vi "PWRVT_Multi_thread.vi"() -> ()   [LabVIEW 2017]
doc: "Use this template to build a producer/consumer design pattern. Use this template when you need to execute a process, such as data analysis, when a data source, such as a triggered acquisition, produces data at an uneven rate and you need to execute the process when the data becomes available."
uses:
  ModbusRTU/Process/Process.lvclass
  ModbusRTU/Caculator/Caculator.lvclass
  ModbusRTU/LNAX301/LNAX301.lvclass
  ModbusRTU/ModbusRTUCmd.ctl
  ModbusRTU/Process/Process.ctl
  ModbusRTU/Caculator/Caculator.ctl
  DLL/Modbus.dll
panel:
  out "connect":bool
  in  "switch":bool
  in  "Debug":bool
  in  "stop":bool
  in  "Tab Control":enum32{"Main", "OA"}(tab)
  out "COM Port":string
  out "Waveform Graph":waveform(dbl)[](graph)
  out "SN":string
  in  "HPF enable":bool
  in  "軸向選擇":enum16{"X", "Y", "Z"}(ring)=enum."Z"
  out "X-Axis Peak(Vel)":dbl
  out "Y-Axis Peak(Vel)":dbl
  out "Z-Axis Peak(Vel)":dbl
  out "X-Axis RMS(Vel)":dbl
  out "Y-Axis RMS(Vel)":dbl
  out "Z-Axis RMS(Vel)":dbl
  out "X-Axis CF(ACC)":dbl
  out "Y-Axis CF(ACC)":dbl
  out "Z-Axis CF(ACC)":dbl
  out "X-Axis RMS(ACC)":dbl
  out "Y-Axis RMS(ACC)":dbl
  out "Z-Axis RMS(ACC)":dbl
  out "X-Axis Peak(ACC)":dbl
  out "Y-Axis Peak(ACC)":dbl
  out "Z-Axis Peak(ACC)":dbl
  out "Z-Axis CF(Vel)":dbl
  out "Y-Axis CF(Vel)":dbl
  out "X-Axis CF(Vel)":dbl
  out "error out 2":errorcluster
  in  "Serial Setting":T1={"baudRate"=3000000, "parity"=0, "dataBits"=8, "stopBits"=1} {"stopBits" items=["None", "One", "Two", "OnePointFive"]; "parity" items=["None", "Odd", "Even", "Mark", "Space"]}
  in  "SR":u16=7812
  # "OA Mode"
  # "Timewave Mode"
  # "HPF:需再開始量測前就決定是否開啟"
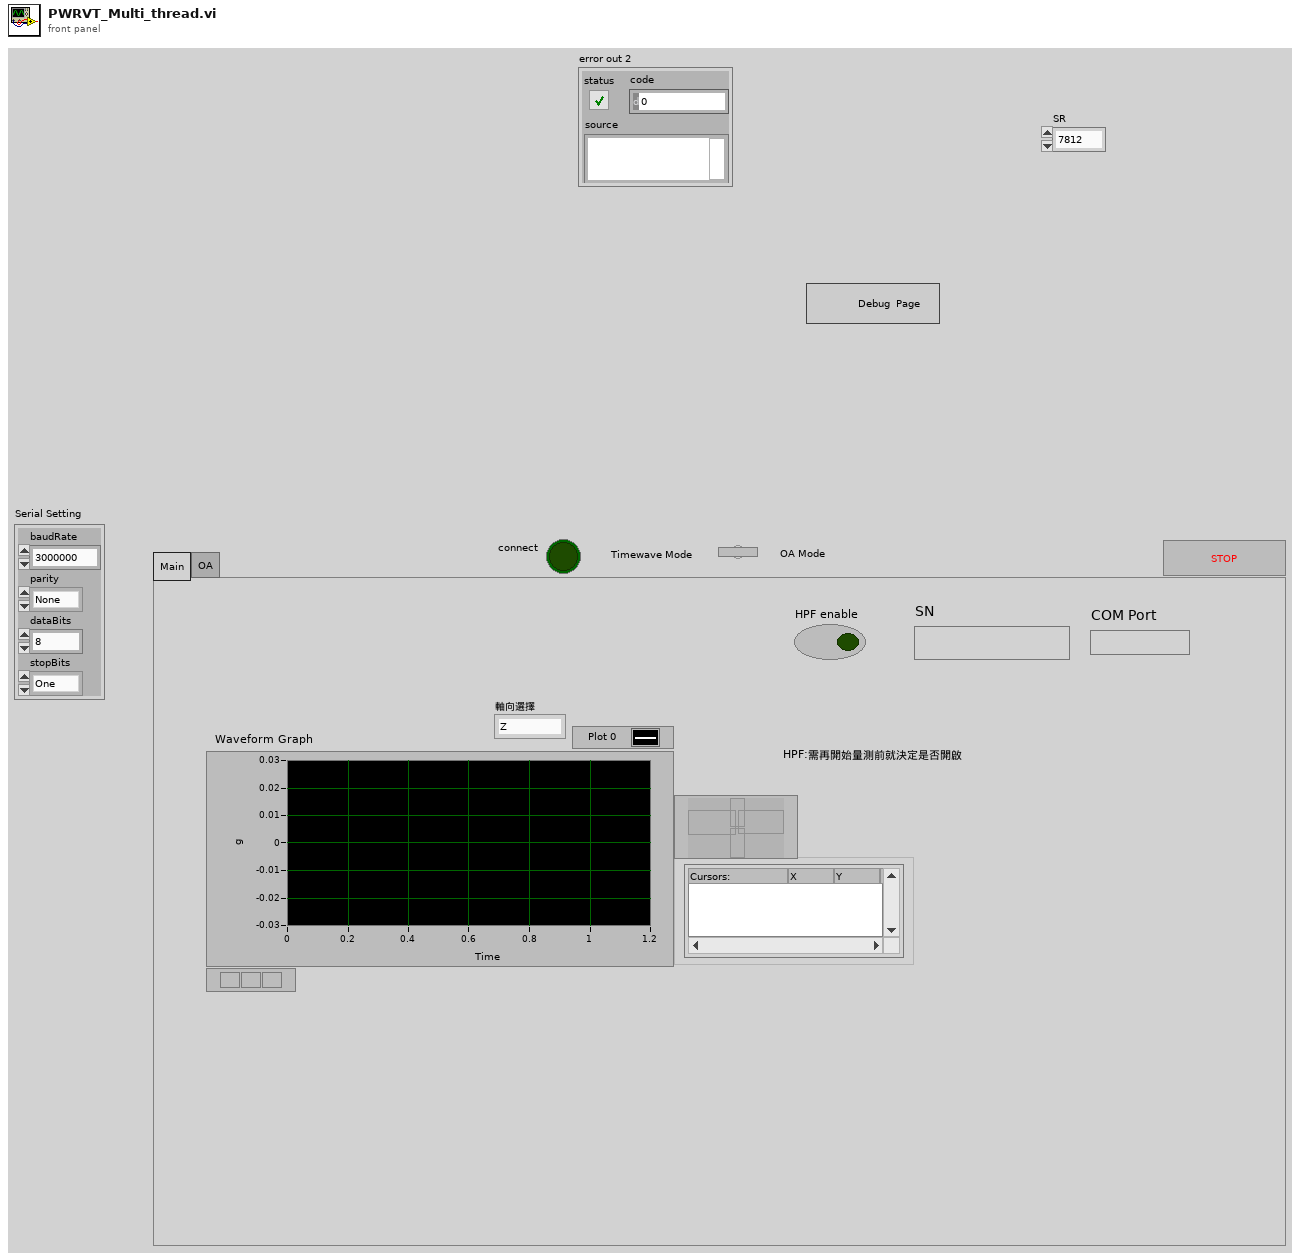
[diagram p1: front panel]
types:
  T1 = cluster{"baudRate":i32, "parity":i32, "dataBits":i32, "stopBits":i32}
  T2 = typedef "MEMS.ctl" = cluster{"LNAX301":refnum<queue>, "Process":refnum<queue>, "Caculator":refnum<queue>}
  T3 = typedef "ModbusRTUCmd.ctl" = cluster{"CMD":enum16{"Idle", "ini", "Connect", "Setup", "Read", "Disconnect", "Exit"}, "Var":variant}
  T4 = typedef "Process.ctl" = cluster{"cmd":enum16{"Idle", "ini", "CheckData", "Disconnect", "UpdateSetup", "UpdateInstance", "Exit"}, "Var":variant}
  T5 = enum16{"Idle", "ini", "Connect", "Setup", "Read", "Disconnect", "Exit"}
  T6 = enum16{"Idle", "ini", "CheckData", "Disconnect", "UpdateSetup", "UpdateInstance", "Exit"}
  T7 = typedef "Caculator.ctl" = cluster{"cmd":enum16{"Idle", "ini", "Disconnect", "UpdateSetup", "ChangeView", "Caculator", "Exit"}, "Var":variant}
  T8 = enum16{"Idle", "ini", "Disconnect", "UpdateSetup", "ChangeView", "Caculator", "Exit"}
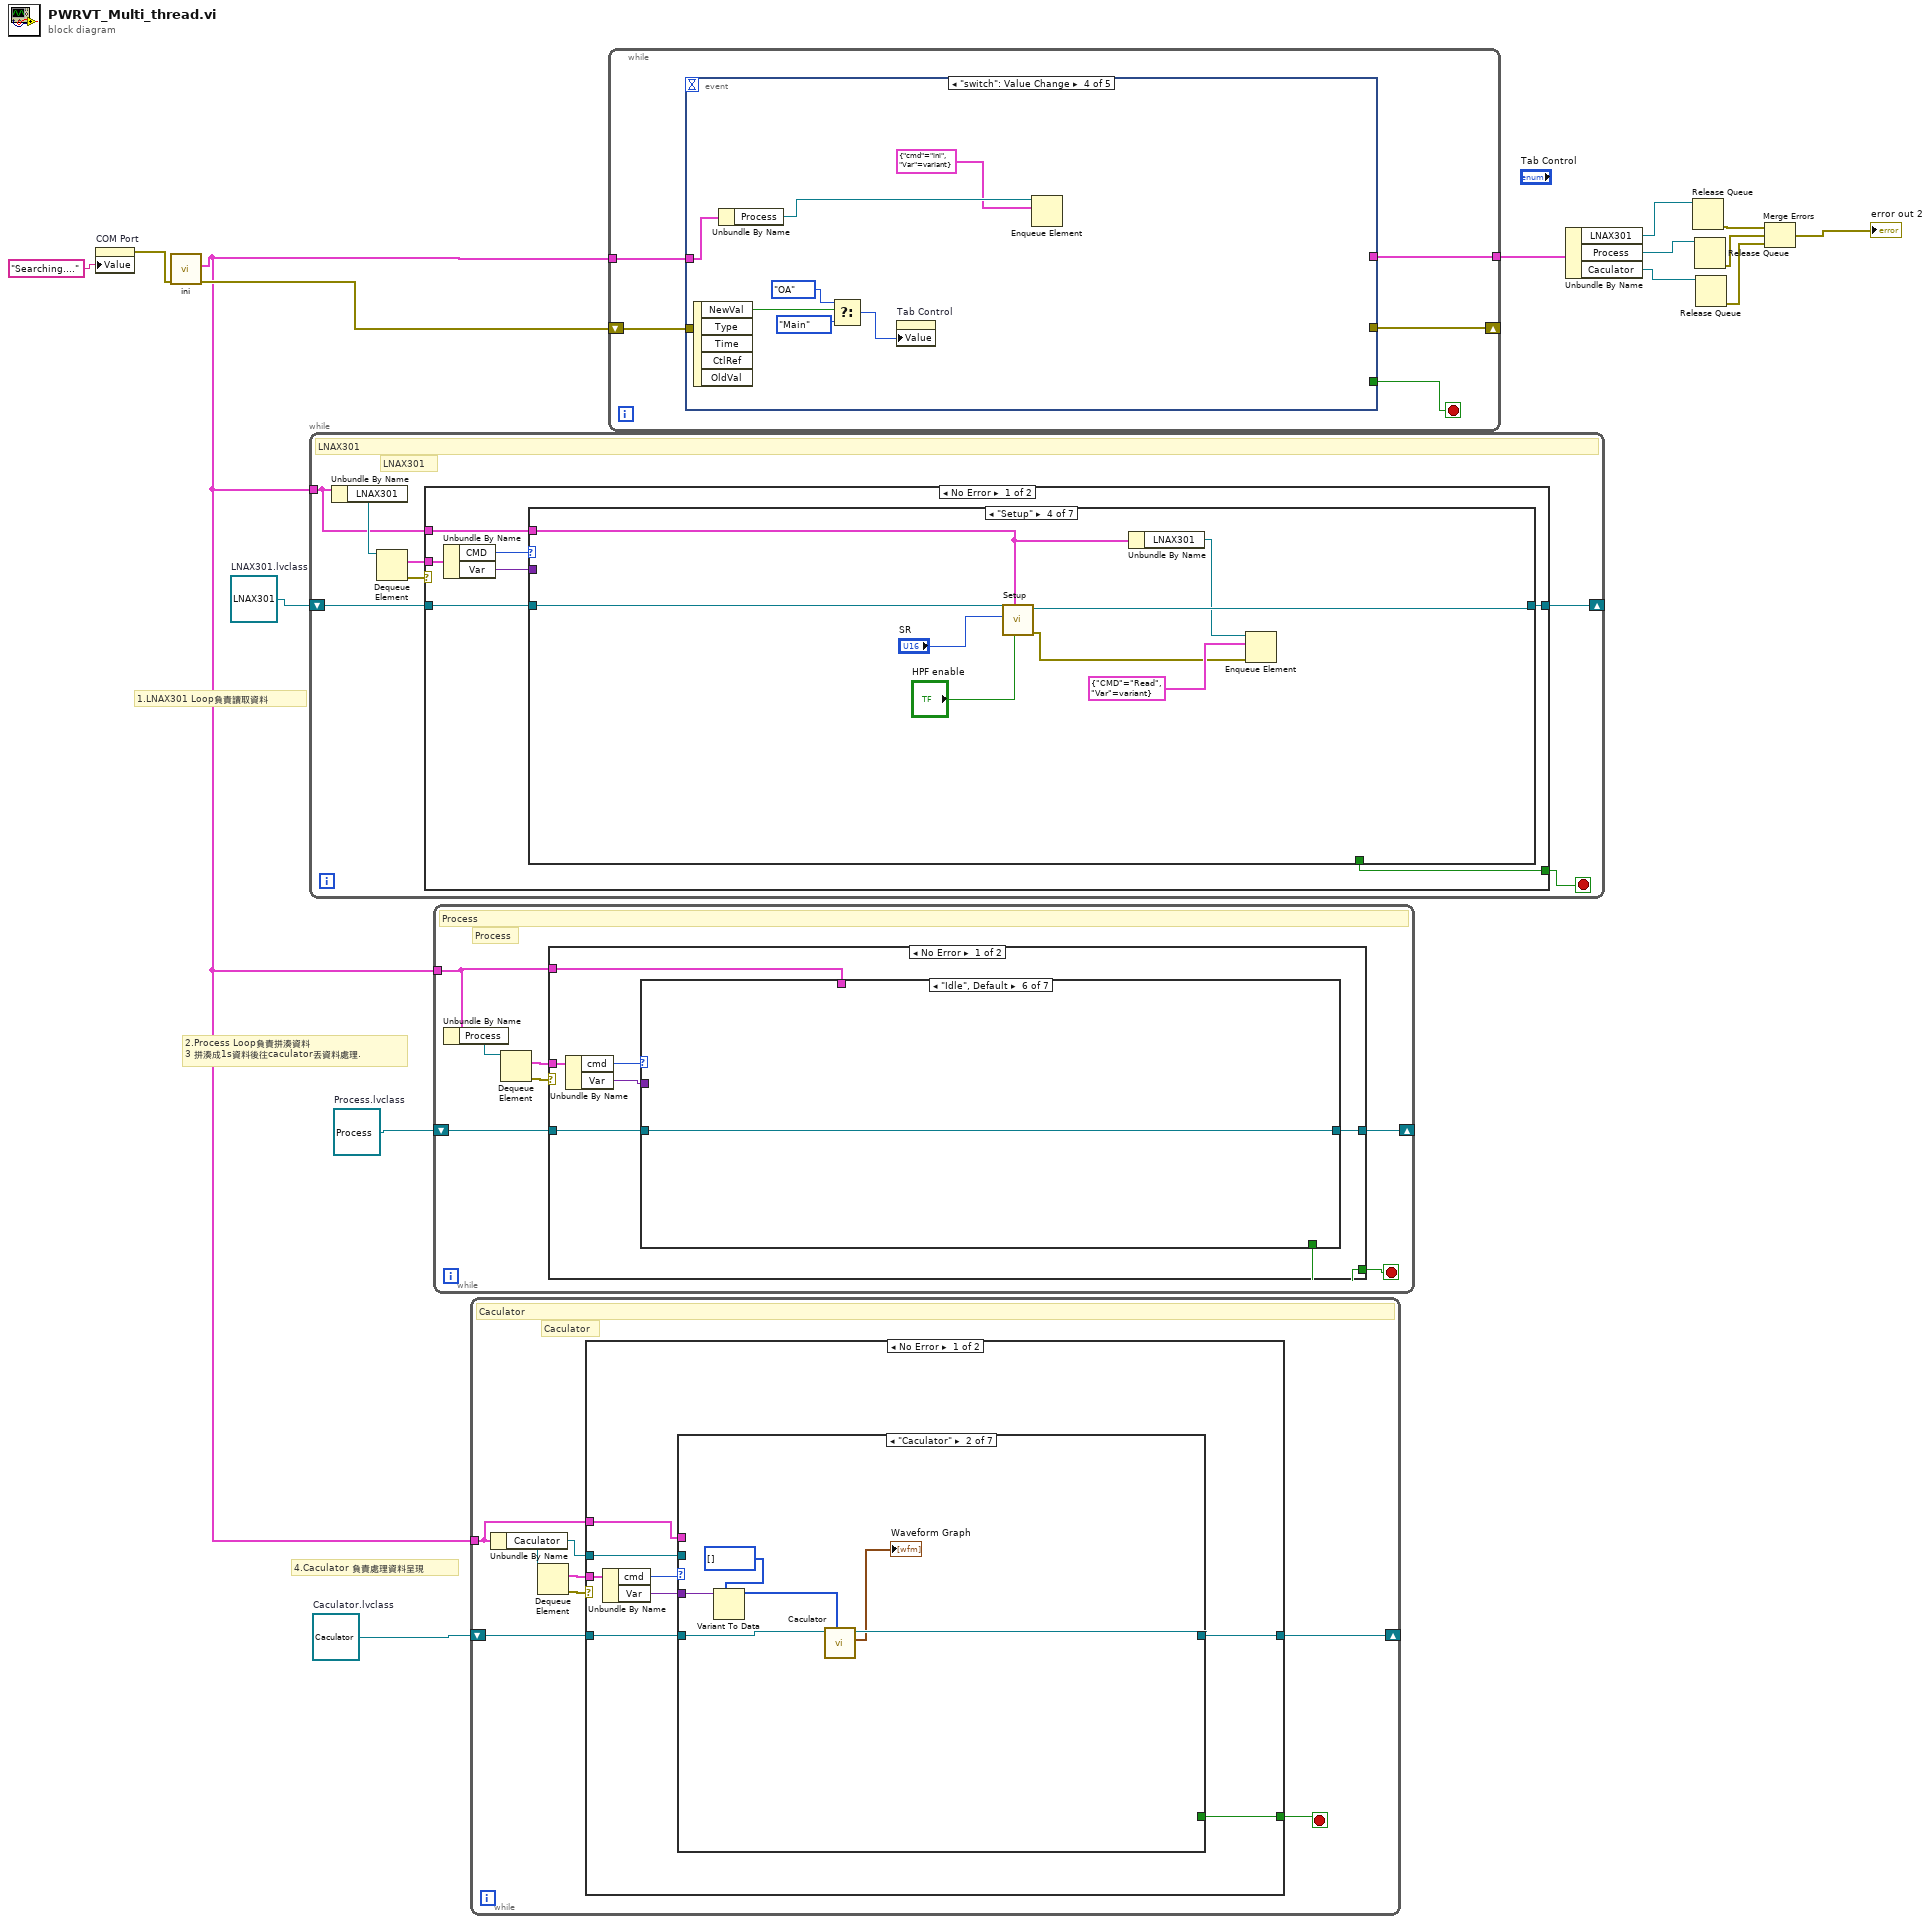
[diagram p0: block diagram]
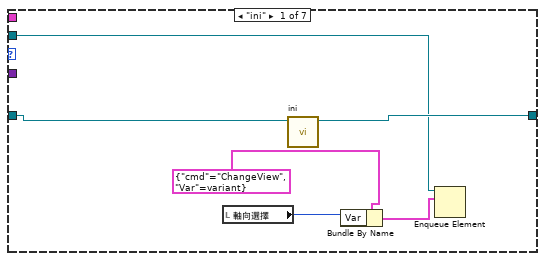
[diagram p2: hidden frame]
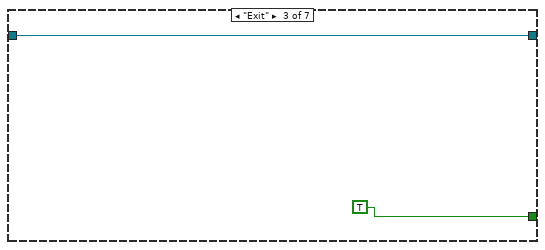
[diagram p3: hidden frame]
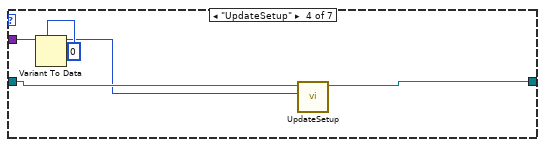
[diagram p4: hidden frame]
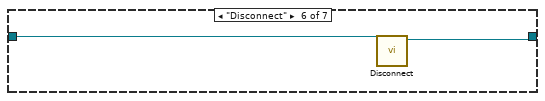
[diagram p6: hidden frame]
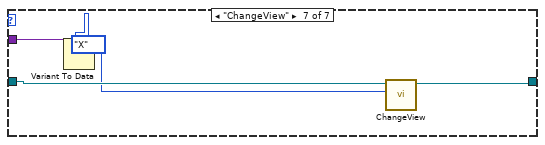
[diagram p7: hidden frame]
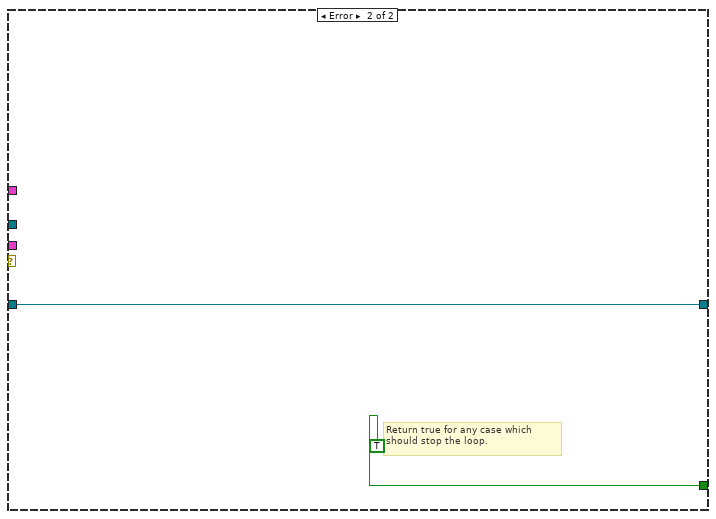
[diagram p8: hidden frame]
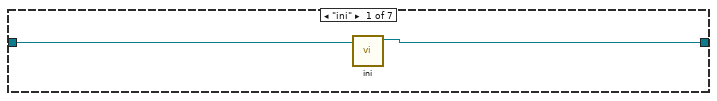
[diagram p9: hidden frame]
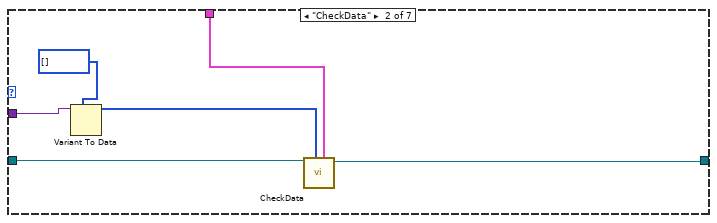
[diagram p10: hidden frame]
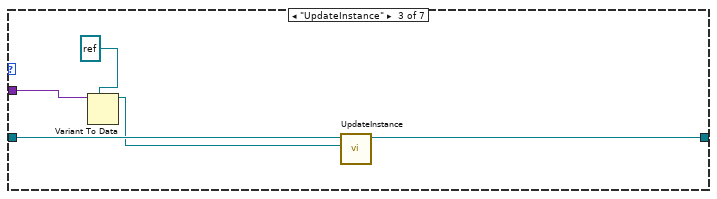
[diagram p11: hidden frame]
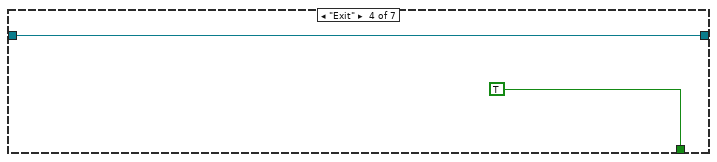
[diagram p12: hidden frame]
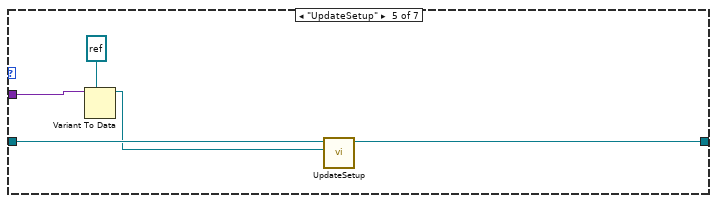
[diagram p13: hidden frame]
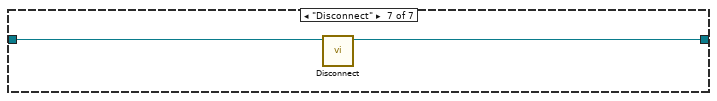
[diagram p14: hidden frame]
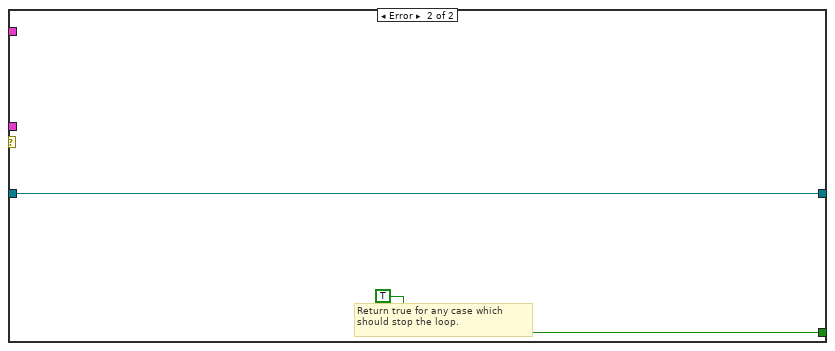
[diagram p15: hidden frame]
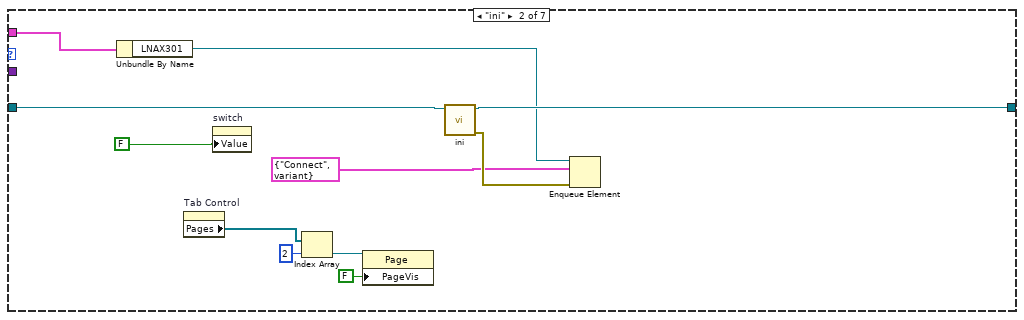
[diagram p17: hidden frame]
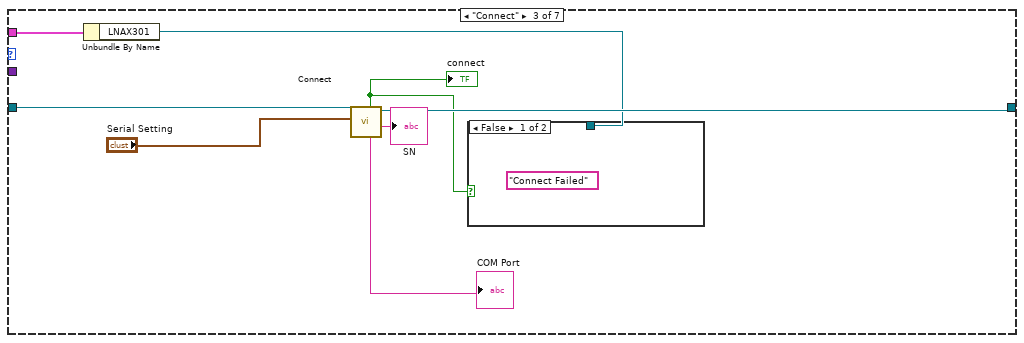
[diagram p18: hidden frame]
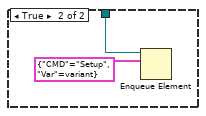
[diagram p19: hidden frame]
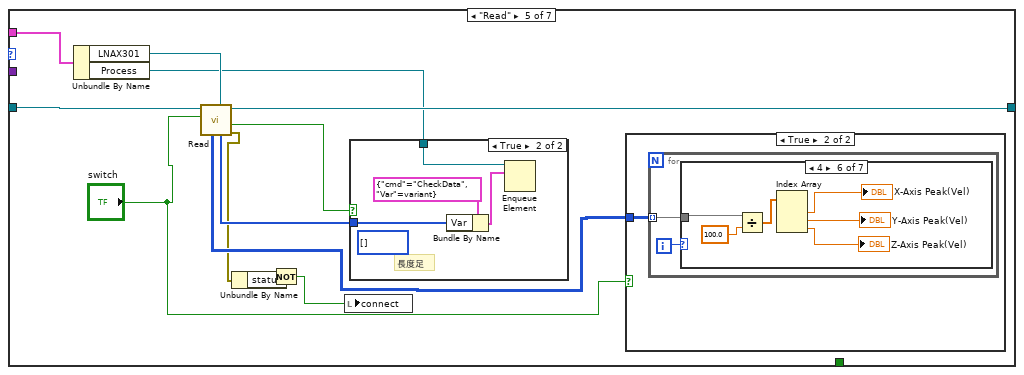
[diagram p20: hidden frame]
diagram:
  w1 = refnum<class "LNAX301.lvclass"> refnum  # LNAX301.lvclass
  w13 = refnum<class "Caculator.lvclass"> refnum  # Caculator.lvclass
  w14 = refnum<class "Process.lvclass"> refnum  # Process.lvclass
  # "4.Caculator 負責處理資料呈現"
  # "2.Process Loop負責拼湊資料\n3 拼湊成1s資料後往caculator丟資料處理."
  # "1.LNAX301 Loop負責讀取資料"
  n1 = property on="COM Port" class="Str"("Value"="Searching...." ("COM Port")) -> (error out=w2:errorcluster)  [unwired: 2 in, 1 out]
  n2 = call "ini.vi"("error in (no error)"=w2) -> ("error out"=w15:errorcluster, "Queue Cluster"=w5:T2)  [unwired: 9 in]
  n3 = while {
    tunnel: w5 -> [w16]
    shift-right: [w17] -> _
    shift-left: w1 -> [w18]
    stop <- w20 stop-if-true
    # "LNAX301"
    # "LNAX301"
    n4 = Unbundle By Name(w16) -> ("LNAX301"=w19:refnum<queue>)
    n5 = Dequeue Element(queue=w19) -> (element=w21:T3, error out=w22:errorcluster)  [unwired: 2 in, 2 out]
    n6 = case shown="No Error" w22 {
      tunnel: w21 -> [w29 _]
      tunnel: [w23 TRUE] -> w20
      tunnel: w18 -> [w26 w121]
      tunnel: [w25 w121] -> w17
      tunnel: w16 -> [w24 _]
      frame No Error {
        n7 = Unbundle By Name(w29) -> ("CMD"=w28:T5, "Var"=w27:variant)
        n8 = case shown="\"Setup\"" w28 {
          tunnel: w27 -> [_ _ _ _ _ _ _]
          tunnel: w26 -> [w30 w41 w49 w52 w71 w117 w120]
          tunnel: [w30 w40 w48 w59 w69 w116 w119] -> w25
          tunnel: w24 -> [_ w38 w46 w55 w70 _ _]
          tunnel: [_ _ _ _ _ _ TRUE] -> w23
          frame "Idle", Default {
          }
          frame "ini" {
            n9 = Unbundle By Name(w38) -> ("LNAX301"=w37:refnum<queue>)
            n10 = property on="Tab Control" class="TabCtl (strict)"() -> ("Pages"=w33:refnum<vi>[])  [unwired: 2 in, 2 out]
            n11 = property on="switch" class="Bool (strict)"("Value"=FALSE ("switch")) -> ()  [unwired: 2 in, 2 out]
            n12 = Index Array(array=w33, index=2) -> (element=w34:refnum<vi>)
            n13 = property class="Page"(reference=w34, "PageVis"=FALSE ("Page Visible")) -> ()  [unwired: 1 in, 2 out]
            n14 = call-dynamic "ini.vi"("LNAX301 in"=w41) -> ("error out"=w39:errorcluster, "LNAX301 out"=w40:refnum<class "LNAX301.lvclass">)  [unwired: 9 in]
            n15 = Enqueue Element(queue=w37, element=T3 {"CMD"=enum."Connect", "Var"=variant}, error in (no error)=w39) -> ()  [unwired: 1 in, 3 out]
          }
          frame "Connect" {
            n16 = Unbundle By Name(w46) -> ("LNAX301"=w45:refnum<queue>)
            n17 = call-dynamic "Connect.vi"("Serial Setting"="Serial Setting", "LNAX301 in"=w49) -> ("SN"=→"SN":string, "LNAX301 out"=w48:refnum<class "LNAX301.lvclass">, "COM Port 2"=→"COM Port":string, "connect"=w47:bool)  [unwired: 5 in, 1 out]
            "connect" <- w47
            n18 = case shown="False" w47 {
              tunnel: w45 -> [_ w51]
              frame False {
                (unwired) "Connect Failed" ("Msg")
              }
              frame True {
                n19 = Enqueue Element(queue=w51, element=T3 {"CMD"=enum."Setup", "Var"=variant}) -> ()  [unwired: 2 in, 3 out]
              }
            }
          }
          frame "Setup" {
            n20 = call-dynamic "Setup.vi"("HPF enable"="HPF enable", "Queue Cluster"=w55, "SR"="SR", "LNAX301 in"=w52) -> ("error out"=w54:errorcluster, "LNAX301 out"=w59:refnum<class "LNAX301.lvclass">)  [unwired: 6 in]
            n21 = Unbundle By Name(w55) -> ("LNAX301"=w58:refnum<queue>)
            n22 = Enqueue Element(queue=w58, element=T3 {"CMD"=enum."Read", "Var"=variant}, error in (no error)=w54) -> ()  [unwired: 1 in, 3 out]
          }
          frame "Read" {
            n23 = Unbundle By Name(w70) -> ("LNAX301"=w64:refnum<queue>, "Process"=w63:refnum<queue>)
            n24 = call-dynamic "Read.vi"("LNAX301"=w64, "Switch Mode"="switch", "LNAX301 in"=w71) -> ("error out"=w60:errorcluster, "Data  ok"=w67:bool, "LNAX301 out"=w69:refnum<class "LNAX301.lvclass">, "data"=w68:i16[], "OA"=w62:i16[][])  [unwired: 3 in, 1 out]
            n25 = Unbundle By Name(w60) -> ("status"=w66:bool)
            n26 = Not(x=w66) -> (.not. x?=w65:bool)
            n27 = local write "connect"(w65) -> ()
            n28 = case shown="True" w67 {
              tunnel: w63 -> [_ w75]
              tunnel: w68 -> [_ w73]
              frame False {
                # "長度足不足124"
              }
              frame True {
                (unwired) i16[] [] ("data")
                # "長度足"
                n29 = Bundle By Name(cluster=T4 {"cmd"=enum."CheckData", "Var"=variant} ("element"), "Var"=w73) -> (w72:T4)
                n30 = Enqueue Element(queue=w75, element=w72) -> ()  [unwired: 2 in, 3 out]
              }
            }
            n31 = case shown="True" "switch" {
              tunnel: w62 -> [_ w76]
              frame False {
              }
              frame True {
                n32 = for {
                  tunnel: w76 -> [w77] mode=indexing
                  i -> [w78]
                  n33 = case shown="4" w78 {
                    tunnel: w77 -> [_ w84 w88 w94 w100 w106 w112]
                    frame Default {
                    }
                    frame 0 {
                      n34 = Divide(x=w84, y=1000.0) -> (x/y=w82:dbl[])
                      n35 = Index Array(array=w82) -> (element #1=→"X-Axis RMS(ACC)":dbl, element #2=→"Y-Axis RMS(ACC)":dbl, element #3=→"Z-Axis RMS(ACC)":dbl)  [unwired: 3 in]
                    }
                    frame 1 {
                      n36 = Divide(x=w88, y=1000.0) -> (x/y=w89:dbl[])
                      n37 = Index Array(array=w89) -> (element #1=→"X-Axis Peak(ACC)":dbl, element #2=→"Y-Axis Peak(ACC)":dbl, element #3=→"Z-Axis Peak(ACC)":dbl)  [unwired: 3 in]
                    }
                    frame 2 {
                      n38 = Divide(x=w94, y=1000.0) -> (x/y=w95:dbl[])
                      n39 = Index Array(array=w95) -> (element #1=→"X-Axis CF(ACC)":dbl, element #2=→"Y-Axis CF(ACC)":dbl, element #3=→"Z-Axis CF(ACC)":dbl)  [unwired: 3 in]
                    }
                    frame 3 {
                      n40 = Divide(x=w100, y=100.0) -> (x/y=w101:dbl[])
                      n41 = Index Array(array=w101) -> (element #1=→"X-Axis RMS(Vel)":dbl, element #2=→"Y-Axis RMS(Vel)":dbl, element #3=→"Z-Axis RMS(Vel)":dbl)  [unwired: 3 in]
                    }
                    frame 4 {
                      n42 = Divide(x=w106, y=100.0) -> (x/y=w107:dbl[])
                      n43 = Index Array(array=w107) -> (element #1=→"X-Axis Peak(Vel)":dbl, element #2=→"Y-Axis Peak(Vel)":dbl, element #3=→"Z-Axis Peak(Vel)":dbl)  [unwired: 3 in]
                    }
                    frame 5 {
                      n44 = Divide(x=w112, y=1000.0) -> (x/y=w113:dbl[])
                      n45 = Index Array(array=w113) -> (element #1=→"X-Axis CF(Vel)":dbl, element #2=→"Y-Axis CF(Vel)":dbl, element #3=→"Z-Axis CF(Vel)":dbl)  [unwired: 3 in]
                    }
                  }
                }
              }
            }
          }
          frame "Disconnect" {
            n46 = Wait (ms)(milliseconds to wait=u32 100) -> ()  [unwired: 1 out]
            n47 = call-dynamic "Disconnect.vi"("LNAX301 in"=w117) -> ("LNAX301 out"=w116:refnum<class "LNAX301.lvclass">)  [unwired: 9 in, 1 out]
          }
          frame "Exit" {
            n48 = call-dynamic "Exit.vi"("LNAX301 in"=w120) -> ("LNAX301 out"=w119:refnum<class "LNAX301.lvclass">)  [unwired: 9 in, 1 out]
          }
        }
      }
      frame Error {
        # "Return true for any case which should stop the loop."
      }
    }
  }
  n49 = while {
    tunnel: w5 -> [w123]
    shift-right: [w124] -> _
    shift-left: w14 -> [w125]
    stop <- w127 stop-if-true
    # "Process"
    # "Process"
    n50 = Unbundle By Name(w123) -> ("Process"=w126:refnum<queue>)
    n51 = Dequeue Element(queue=w126) -> (element=w128:T4, error out=w129:errorcluster)  [unwired: 2 in, 2 out]
    n52 = case shown="No Error" w129 {
      tunnel: w128 -> [w136 _]
      tunnel: [w130 TRUE] -> w127
      tunnel: w125 -> [w133 w160]
      tunnel: [w132 w160] -> w124
      tunnel: w123 -> [w131 _]
      frame No Error {
        n53 = Unbundle By Name(w136) -> ("cmd"=w135:T6, "Var"=w134:variant)
        n54 = case shown="\"Idle\", Default" w135 {
          tunnel: w134 -> [_ w144 w147 _ w154 _ _]
          tunnel: w133 -> [w138 w143 w149 w151 w156 w157 w159]
          tunnel: [w137 w142 w148 w151 w155 w157 w158] -> w132
          tunnel: w131 -> [_ w141 _ _ _ _ _]
          tunnel: [_ _ _ TRUE _ _ _] -> w130
          frame "ini" {
            n55 = call-dynamic "ini.vi"("Process in"=w138) -> ("Process out"=w137:refnum<class "Process.lvclass">)  [unwired: 9 in, 1 out]
          }
          frame "CheckData" {
            n56 = Variant To Data(type=i16[] [] ("data"), Variant=w144) -> (data=w139:i16[])  [unwired: 1 in, 1 out]
            n57 = call-dynamic "CheckData.vi"("Queue Cluster"=w141, "DATA"=w139, "Process in"=w143) -> ("Process out"=w142:refnum<class "Process.lvclass">)  [unwired: 7 in, 1 out]
          }
          frame "UpdateInstance" {
            n58 = Variant To Data(type=refnum<k24> refnum (".NET Refnum out"), Variant=w147) -> (data=w146:refnum<k24>)  [unwired: 1 in, 1 out]
            n59 = call-dynamic "UpdateInstance.vi"(".NET Refnum"=w146, "Process in"=w149) -> ("Process out"=w148:refnum<class "Process.lvclass">)  [unwired: 8 in, 1 out]
          }
          frame "Exit" {
          }
          frame "UpdateSetup" {
            n60 = Variant To Data(type=refnum<k24> refnum (".NET Refnum"), Variant=w154) -> (data=w153:refnum<k24>)  [unwired: 1 in, 1 out]
            n61 = call-dynamic "UpdateSetup.vi"(".NET Refnum"=w153, "Process in"=w156) -> ("Process out"=w155:refnum<class "Process.lvclass">)  [unwired: 8 in, 1 out]
          }
          frame "Idle", Default {
          }
          frame "Disconnect" {
            n62 = call-dynamic "Disconnect.vi"("Process in"=w159) -> ("Process out"=w158:refnum<class "Process.lvclass">)  [unwired: 9 in, 1 out]
          }
        }
      }
      frame Error {
        # "Return true for any case which should stop the loop."
      }
    }
  }
  n63 = while {
    tunnel: w5 -> [w163]
    shift-right: [w164] -> _
    shift-left: w13 -> [w165]
    stop <- w166 stop-if-true
    # "Caculator"
    # "Caculator"
    n64 = Unbundle By Name(w163) -> ("Caculator"=w162:refnum<queue>)
    n65 = Dequeue Element(queue=w162) -> (element=w167:T7, error out=w168:errorcluster)  [unwired: 2 in, 2 out]
    n66 = case shown="No Error" w168 {
      tunnel: w167 -> [w176 _]
      tunnel: [w172 TRUE] -> w166
      tunnel: w165 -> [w174 w204]
      tunnel: [w173 w204] -> w164
      tunnel: w163 -> [w171 _]
      tunnel: w162 -> [w170 _]
      frame No Error {
        n67 = Unbundle By Name(w176) -> ("cmd"=w169:T8, "Var"=w175:variant)
        n68 = case shown="\"Caculator\"" w169 {
          tunnel: w175 -> [_ w187 _ w194 _ _ w201]
          tunnel: w174 -> [w182 w186 w190 w193 w196 w198 w203]
          tunnel: [w181 w185 w190 w192 w196 w197 w202] -> w173
          tunnel: [_ _ TRUE _ _ _ _] -> w172
          tunnel: w171 -> [_ _ _ _ _ _ _]
          tunnel: w170 -> [w178 _ _ _ _ _ _]
          frame "ini" {
            n69 = local read "軸向選擇"() -> (w177:enum16{"X", "Y", "Z"})
            n70 = call-dynamic "ini.vi"("Caculator in"=w182) -> ("Caculator out"=w181:refnum<class "Caculator.lvclass">)  [unwired: 9 in, 1 out]
            n71 = Bundle By Name(cluster=T7 {"cmd"=enum."ChangeView", "Var"=variant} ("element"), "Var"=w177) -> (w179:T7)
            n72 = Enqueue Element(queue=w178, element=w179) -> ()  [unwired: 2 in, 3 out]
          }
          frame "Caculator" {
            n73 = Variant To Data(type=i16[] [] ("register values"), Variant=w187) -> (data=w184:i16[])  [unwired: 1 in, 1 out]
            n74 = call-dynamic "Caculator.vi"("DATA"=w184, "Caculator in"=w186) -> ("Waveform Graph"=→"Waveform Graph":waveform(dbl)[], "Caculator out"=w185:refnum<class "Caculator.lvclass">)  [unwired: 7 in, 1 out]
          }
          frame "Exit" {
          }
          frame "UpdateSetup" {
            n75 = Variant To Data(type=u16 0 ("SR"), Variant=w194) -> (data=w191:u16)  [unwired: 1 in, 1 out]
            n76 = call-dynamic "UpdateSetup.vi"("data"=w191, "Caculator in"=w193) -> ("Caculator out"=w192:refnum<class "Caculator.lvclass">)  [unwired: 8 in, 1 out]
          }
          frame "Idle", Default {
          }
          frame "Disconnect" {
            n77 = call-dynamic "Disconnect.vi"("Caculator in"=w198) -> ("Caculator out"=w197:refnum<class "Caculator.lvclass">)  [unwired: 9 in, 1 out]
          }
          frame "ChangeView" {
            n78 = Variant To Data(type=enum16{"X", "Y", "Z"}."X" ("NewVal"), Variant=w201) -> (data=w199:enum16{"X", "Y", "Z"})  [unwired: 1 in, 1 out]
            n79 = call-dynamic "ChangeView.vi"("AxisView"=w199, "Caculator in"=w203) -> ("Caculator out"=w202:refnum<class "Caculator.lvclass">)  [unwired: 8 in, 1 out]
          }
        }
      }
      frame Error {
        # "Return true for any case which should stop the loop."
      }
    }
  }
  n80 = while {
    shift-right: [w209] -> _
    shift-left: w15 -> [w210]
    tunnel: w5 -> [w206]
    tunnel: [w207] -> w12
    stop <- w208 stop-if-true
    n81 = event shown="[3] \"switch\": Value Change" {
      selector: _ -> [_ _ _ _ _]
      dyn-events: _ -> [_ _ _ _ _]
      timeout: _ -> [_ _ _ _ _]
      tunnel: w210 -> [w212 _ _ _ _]
      tunnel: [w212 w213 _ _ _] -> w209
      tunnel: [_ "stop" _ _ _] -> w208
      tunnel: [w211 _ _ _ w270] -> w207
      tunnel: w206 -> [w211 w230 w262 w265 w270]
      event Timeout {
        n82 = event-data() -> ()  [unwired: 1 in, 3 out]
      }
      event "stop": Value Change {
        n83 = event-data() -> ()  [unwired: 1 in, 1 out]
        n84 = Unbundle By Name(w230) -> ("LNAX301"=w229:refnum<queue>, "Process"=w235:refnum<queue>, "Caculator"=w234:refnum<queue>)
        n85 = Flush Queue(queue=w229) -> (queue out=w228:refnum<queue>, error out=w227:errorcluster)  [unwired: 1 in, 1 out]
        n86 = Enqueue Element(queue=w234, element=T7 {"cmd"=enum."Disconnect", "Var"=variant}) -> (queue out=w223:refnum<queue>, error out=w224:errorcluster)  [unwired: 2 in, 1 out]
        n87 = Enqueue Element(queue=w235, element=T4 {"cmd"=enum."Disconnect", "Var"=variant}) -> (queue out=w225:refnum<queue>, error out=w226:errorcluster)  [unwired: 2 in, 1 out]
        n88 = Enqueue Element(queue=w228, element=T3 {"CMD"=enum."Disconnect", "Var"=variant}, error in (no error)=w227) -> (queue out=w237:refnum<queue>, error out=w236:errorcluster)  [unwired: 1 in, 1 out]
        n89 = flat-sequence {
          tunnel: w223 -> [w240]
          tunnel: w224 -> [w241]
          tunnel: w225 -> [w242]
          tunnel: w226 -> [w243]
          tunnel: w236 -> [w244]
          tunnel: w237 -> [w245]
          tunnel: [w245] -> w222
          tunnel: [w244] -> w221
          tunnel: [w243] -> w220
          tunnel: [w242] -> w219
          tunnel: [w241] -> w218
          tunnel: [w240] -> w217
          tunnel: w222 -> [w257]
          tunnel: w221 -> [w256]
          tunnel: w220 -> [w254]
          tunnel: w219 -> [w253]
          tunnel: w218 -> [w252]
          tunnel: w217 -> [w251]
          tunnel: [w248] -> w216
          tunnel: [w247] -> w215
          tunnel: [w246] -> w214
          frame #0 {
            n90 = Wait (ms)(milliseconds to wait=u32 100) -> ()  [unwired: 1 out]
          }
          frame #1 {
            n91 = Enqueue Element(queue=w251, element=T7 {"cmd"=enum."Exit", "Var"=variant}, error in (no error)=w252) -> (error out=w248:errorcluster)  [unwired: 1 in, 2 out]
            n92 = Enqueue Element(queue=w257, element=T3 {"CMD"=enum."Exit", "Var"=variant}, error in (no error)=w256) -> (error out=w246:errorcluster)  [unwired: 1 in, 2 out]
            n93 = Enqueue Element(queue=w253, element=T4 {"cmd"=enum."Exit", "Var"=variant}, error in (no error)=w254) -> (error out=w247:errorcluster)  [unwired: 1 in, 2 out]
          }
        }
        n94 = Merge Errors(w214, w215, w216) -> (w213:errorcluster)
      }
      event "軸向選擇": Value Change {
        # "X:0\nY:1\nZ:2"
        n95 = event-data() -> ("NewVal"=w258:enum16{"X", "Y", "Z"})  [unwired: 1 in]
        n96 = Unbundle By Name(w262) -> ("Caculator"=w261:refnum<queue>)
        n97 = Bundle By Name(cluster=T7 {"cmd"=enum."ChangeView", "Var"=variant} ("element"), "Var"=w258) -> (w259:T7)
        n98 = Enqueue Element(queue=w261, element=w259) -> ()  [unwired: 2 in, 3 out]
      }
      event "switch": Value Change {
        n99 = event-data() -> ("NewVal"=w269:bool)  [unwired: 1 in, 4 out]
        n100 = Unbundle By Name(w265) -> ("Process"=w264:refnum<queue>)
        n101 = Select(t=enum32{"Main", "OA", "Debug"}."OA" ("Tab Control"), s=w269, f=enum32{"Main", "OA", "Debug"}."Main" ("Tab Control")) -> (s? t:f=w266:enum32{"Main", "OA", "Debug"})
        n102 = property on="Tab Control" class="TabCtl (strict)"("Value"=w266) -> ()  [unwired: 2 in, 2 out]
        n103 = Enqueue Element(queue=w264, element=T4 {"cmd"=enum."ini", "Var"=variant}) -> ()  [unwired: 2 in, 3 out]
      }
      event "Debug": Value Change {
        n104 = event-data() -> ("NewVal"=w271:bool)  [unwired: 1 in, 4 out]
        n105 = property on="Tab Control" class="TabCtl (strict)"() -> ("Pages"=w274:refnum<vi>[])  [unwired: 2 in, 2 out]
        n106 = Index Array(array=w274, index=2) -> (element=w272:refnum<vi>)
        n107 = property class="Page"(reference=w272, "PageVis"=w271) -> ()  [unwired: 1 in, 2 out]
      }
    }
  }
  n108 = Unbundle By Name(w12) -> ("LNAX301"=w11:refnum<queue>, "Process"=w10:refnum<queue>, "Caculator"=w9:refnum<queue>)
  n109 = Release Queue(queue=w11) -> (error out=w8:errorcluster)  [unwired: 2 in, 2 out]
  n110 = Release Queue(queue=w10) -> (error out=w7:errorcluster)  [unwired: 2 in, 2 out]
  n111 = Release Queue(queue=w9) -> (error out=w6:errorcluster)  [unwired: 2 in, 2 out]
  n112 = Merge Errors(w8, w7, w6) -> (→"error out 2":errorcluster)
